vi "Test Parse Request.vi"(8 "error in (no error)":errorcluster) -> (0 "error out":errorcluster)   [LabVIEW 2016]
uses:
  Response/Response.lvclass
  <vilib>/addons/_JKI Toolkits/Caraya/classes/Test/Test.lvclass
  <vilib>/addons/_JKI Toolkits/Caraya/classes/Assert/Assert.lvclass
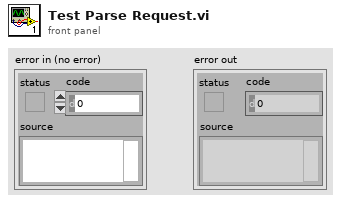
[diagram p1: front panel]
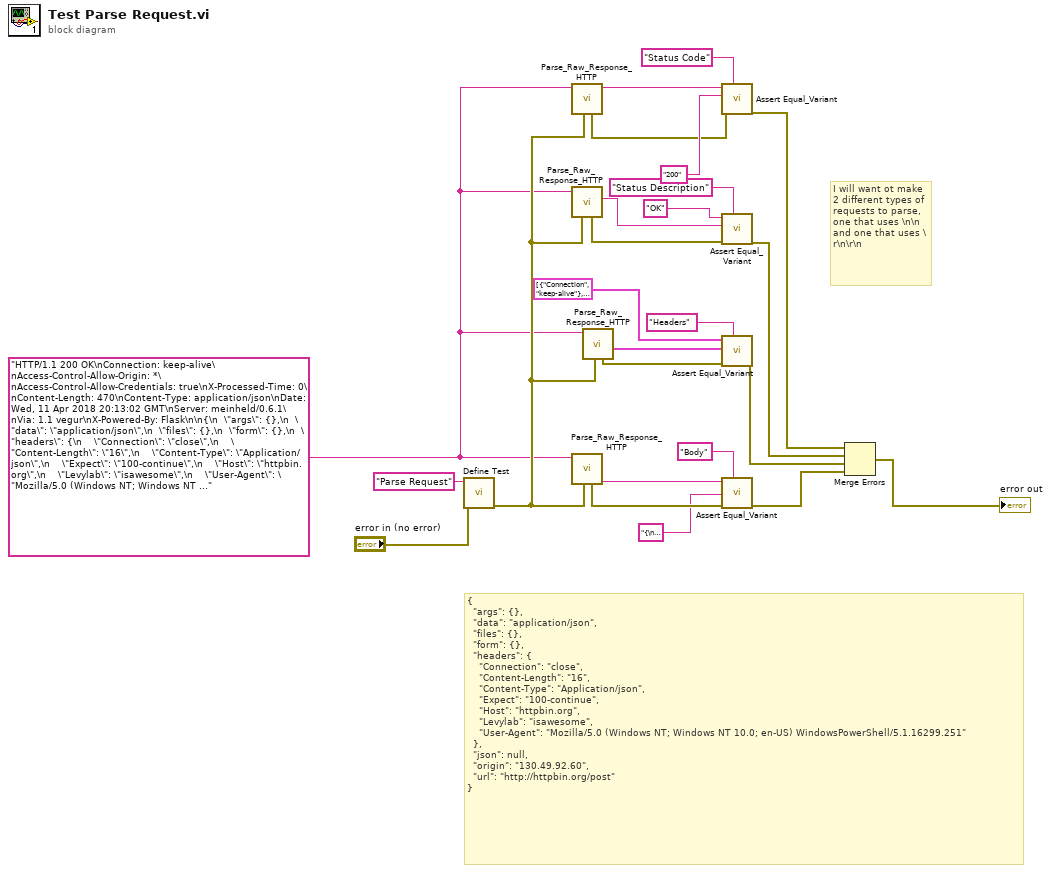
[diagram p0: block diagram]
diagram:
  w10 = "HTTP/1.1 200 OK\nConnection: keep-alive\nAccess-Control-Allow-Origin: *\nAccess-Control-Allow-Credentials: true\nX-Processed-Time: 0\nContent-Length: 470\nContent-Type: application/json\nDate: Wed, 11 Apr 2018 20:13:02 GMT\nServer: meinheld/0.6.1\nVia: 1.1 vegur\nX-Powered-By: Flask\n\n{\n  \"args\": {},\n  \"data\": \"application/json\",\n  \"files\": {},\n  \"form\": {},\n  \"headers\": {\n    \"Connection\": \"close\",\n    \"Content-Length\": \"16\",\n    \"Content-Type\": \"Application/json\",\n    \"Expect\": \"100-continue\",\n    \"Host\": \"httpbin.org\",\n    \"Levylab\": \"isawesome\",\n    \"User-Agent\": \"Mozilla/5.0 (Windows NT; Windows NT 10.0; en-US) WindowsPowerShell/5.1.16299.251\"\n  },\n  \"json\": null,\n  \"origin\": \"130.49.92.60\",\n  \"url\": \"http://httpbin.org/post\"\n}"
  # "I will want ot make 2 different types of requests to parse, one that uses \\n\\n and one that uses \\r\\n\\r\\n"
  # "{\n  \"args\": {},\n  \"data\": \"application/json\",\n  \"files\": {},\n  \"form\": {},\n  \"headers\": {\n    \"Connection\": \"close\",\n    \"Content-Length\": \"16\",\n    \"Content-Type\": \"Application/json\",\n    \"Expect\": \"100-continue\",\n    \"Host\": \"httpbin.org\",\n    \"Levylab\": \"isawesome\",\n    \"User-Agent\": \"Mozilla/5.0 (Windows NT; Windows NT 10.0; en-US) WindowsPowerShell/5.1.16299.251\"\n  },\n  \"json\": null,\n  \"origin\": \"130.49.92.60\",\n  \"url\": \"http://httpbin.org/post\"\n}"
  n1 = call <vilib>:"Define Test.vi"("error in (no error)"="error in (no error)", "Label (VI Title)"="Parse Request") -> ("error out"=w11:errorcluster)  [unwired: 9 in]
  n2 = call "Parse_Raw_Response_HTTP.vi"("error in (no error)"=w11, "HTTP Response"=w10) -> ("Status Code"=w14:string, "error out"=w7:errorcluster)  [unwired: 5 in, 3 out]
  n3 = call "Parse_Raw_Response_HTTP.vi"("error in (no error)"=w11, "HTTP Response"=w10) -> ("Status Description"=w17:string, "error out"=w13:errorcluster)  [unwired: 5 in, 3 out]
  n4 = call "Parse_Raw_Response_HTTP.vi"("error in (no error)"=w11, "HTTP Response"=w10) -> ("Body"=w21:string, "error out"=w23:errorcluster)  [unwired: 5 in, 3 out]
  n5 = call "Parse_Raw_Response_HTTP.vi"("error in (no error)"=w11, "HTTP Response"=w10) -> ("Headers"=w18:cluster{"Name":string, "Value":string}[], "error out"=w12:errorcluster)  [unwired: 5 in, 3 out]
  n6 = call <vilib>:"Assert Equal_Variant.vi"("Label"="Status Code", "error in (no error)"=w7, "Y"="200", "X"=w14) -> ("error out"=w4:errorcluster)  [unwired: 7 in]
  n7 = call <vilib>:"Assert Equal_Variant.vi"("Label"="Status Description", "error in (no error)"=w13, "Y"=w17, "X"="OK") -> ("error out"=w5:errorcluster)  [unwired: 7 in]
  n8 = call <vilib>:"Assert Equal_Variant.vi"("Label"="Headers", "error in (no error)"=w12, "Y"=w18, "X"=cluster{"Name":string, "Value":string}[] [{"Name"="Connection", "Value"="keep-alive"}, {"Name"="Access-Control-Allow-Origin", "Value"="*"}, {"Name"="Access-Control-Allow-Credentials", "Value"="true"}, {"Name"="X-Processed-Time", "Value"="0"}, {"Name"="Content-Length", "Value"="470"}, {"Name"="Content-Type", "Value"="application/json"}, {"Name"="Date", "Value"="Wed, 11 Apr 2018 20:13:02 GMT"}, {"Name"="Server", "Value"="meinheld/0.6.1"}, {"Name"="Via", "Value"="1.1 vegur"}, {"Name"="X-Powered-By", "Value"="Flask"}] ("Headers")) -> ("error out"=w6:errorcluster)  [unwired: 7 in]
  n9 = call <vilib>:"Assert Equal_Variant.vi"("Label"="Body", "error in (no error)"=w23, "Y"="{\n  \"args\": {},\n  \"data\": \"application/json\",\n  \"files\": {},\n  \"form\": {},\n  \"headers\": {\n    \"Connection\": \"close\",\n    \"Content-Length\": \"16\",\n    \"Content-Type\": \"Application/json\",\n    \"Expect\": \"100-continue\",\n    \"Host\": \"httpbin.org\",\n    \"Levylab\": \"isawesome\",\n    \"User-Agent\": \"Mozilla/5.0 (Windows NT; Windows NT 10.0; en-US) WindowsPowerShell/5.1.16299.251\"\n  },\n  \"json\": null,\n  \"origin\": \"130.49.92.60\",\n  \"url\": \"http://httpbin.org/post\"\n}", "X"=w21) -> ("error out"=w3:errorcluster)  [unwired: 7 in]
  n10 = Merge Errors(w4, w5, w6, w3) -> (→"error out":errorcluster)
